vi "Calibrate Input Data Query.vi"(8 "error in":errorcluster, 10 "Input Channel":i32(ring) caption="Channel" items=["Input Channel 1", "Input Channel 2", "Input Channel 3", "Input Channel 4"], 11 "Instrument Handle In":i32) -> (0 "error out":errorcluster, 1 "Path Gain Code":u16, 2 "Path Offset Code":u16, 3 "Instrument Handle Out":i32)   [LabVIEW 8.6, in "ZTScopeM.lvlib"]
doc: "Query the instrument's input data calibration settings. See the instrument calibration manual for more information."
uses:
  ZTScopeM.lvlib
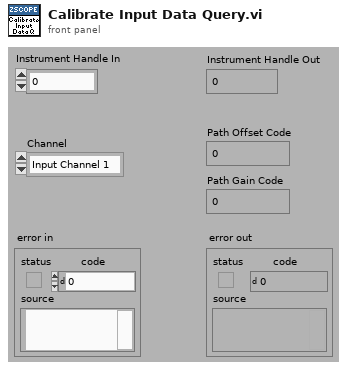
[diagram p1: front panel]
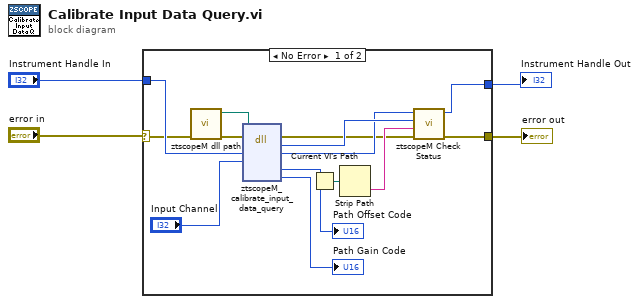
[diagram p0: block diagram]
diagram:
  n1 = case shown="No Error" "error in" {
    selector: "error in" -> [w8 w20]
    tunnel: [w13 w20] -> w1
    tunnel: "Instrument Handle In" -> [w18 w19]
    tunnel: [w12 w19] -> w3
    frame #0 {
      n2 = call "ztscopeM dll path.vi"("error in (no error)"=w8) -> ("error out"=w6:errorcluster, "<instrument>.dll path"=w7:path)  [unwired: 9 in]
      n3 = dll-call lib="C:/Program Files (x86)/National Instruments/LabVIEW 2013/instr.lib/ztscopem/ztscopeM.dll" fn="ztscopeM_calibrate_input_data_query"(path in=w7, error in=w6, "instrumentHandle"=w18, "channel"="Input Channel") -> (error out=w5:errorcluster, w15:i32, "instrumentHandle"=w14:i32, "pathOffsetCode"=→"Path Offset Code":u16, "pathGainCode"=→"Path Gain Code":u16)  [unwired: 4 in, 1 out]
      n4 = Current VI's Path() -> (path=w17:path)
      n5 = Strip Path(path=w17) -> (name=w16:string)  [unwired: 1 out]
      n6 = call "ztscopeM Check Status.vi"("error in"=w5, "name of VI"=w16, "status (return code)"=w15, "instrument handle in"=w14) -> ("error out"=w13:errorcluster, "instrument handle out"=w12:i32)  [unwired: 2 in]
    }
    frame #1 {
    }
  }
  "Instrument Handle Out" <- w3
  "error out" <- w1
